vi "GL SwitchStatus.vi"(6 "error in (no error)":errorcluster, 7 "ShowWarning?":bool, 8 "Axis":T2 items=["Axis 1", "Axis 2", "Axis 3", "Axis 4", "Axis 5", "Axis 6", "Axis 7", "Axis 8"], 9 "Galil.IGalil":refnum<k7>) -> (0 "error out":errorcluster, 1 "TS Status":T1, 2 "Axis Out":T2 items=["Axis 1", "Axis 2", "Axis 3", "Axis 4", "Axis 5", "Axis 6", "Axis 7", "Axis 8"], 3 "ref out":refnum<k7>)   [LabVIEW 2022 SP3]
doc: "Sets the operation mode for an axis or vector space."
uses:
  GL Axis Control.ctl
  Command Menu.ctl
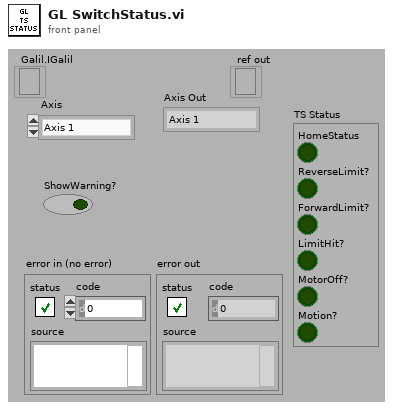
[diagram p1: front panel]
types:
  T1 = cluster{"HomeStatus":bool, "ReverseLimit?":bool, "ForwardLimit?":bool, "LimitHit?":bool, "MotorOff?":bool, "Motion?":bool}
  T2 = typedef "GL Axis Control.ctl" = u16
  T3 = typedef "Command Menu.ctl" = enum16{"CommandPassThrough", "Abort Motion", "Define Pos", "Velocity", "Acceleration", "Deceleration", "Position Rel", "Postion Abs", "Begin Move", "After Move", "Home", "KI", "KD", "KP", "IL", "Config I/O", "Set Bit", "Clear Bit", "Motor Off", "Moto On", "Status", "Execute", "Halt Execute", "HX Status", "Tell Velocity", "Check Motion", "BreakPoint", "Tell Position", "Current Code Line", "Tell Switches", "OC Force On", "OC Off", "Pos Soft Limit", "Rev Soft Limit"}
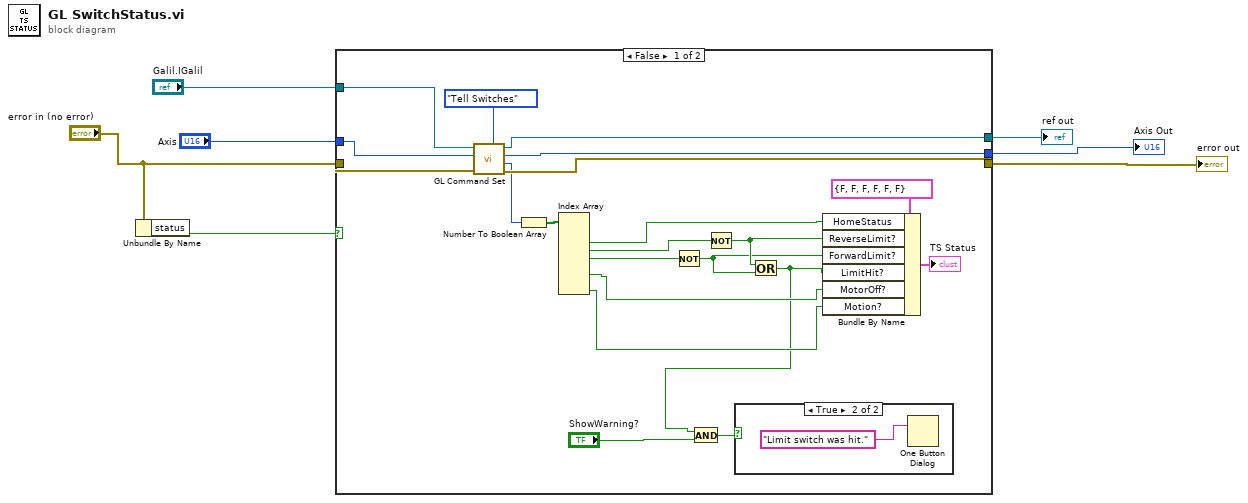
[diagram p0: block diagram]
diagram:
  n1 = Unbundle By Name("error in (no error)") -> ("status"=w5:bool)
  n2 = case shown="False" w5 {
    tunnel: "error in (no error)" -> [w26 w32]
    tunnel: [w28 w32] -> w6
    tunnel: "Galil.IGalil" -> [w14 w31]
    tunnel: "Axis" -> [w13 w30]
    tunnel: [w12 w31] -> w2
    tunnel: [w11 w30] -> w1
    frame False {
      n3 = call "GL Command Set.vi"("Command"=Command_Menu."Tell Switches", "error in (no error)"=w26, "Axis"=w13, "Galil.IGalil"=w14) -> ("error out"=w28:errorcluster, "Response#"=w25:i32, "Axis Out"=w11:T2, "ref out"=w12:refnum<k7>)  [unwired: 3 in, 1 out]
      n4 = Number To Boolean Array(number=w25) -> (Boolean array=w24:bool[])
      n5 = Index Array(array=w24) -> (element #2=w19:bool, element #3=w17:bool, element #4=w15:bool, element #6=w16:bool, element #8=w20:bool)  [unwired: 8 in, 3 out]
      n6 = Not(x=w15) -> (.not. x?=w21:bool)
      n7 = Not(x=w17) -> (.not. x?=w22:bool)
      n8 = Or(x=w22, y=w21) -> (x .or. y?=w10:bool)
      n9 = And(x=w10, y="ShowWarning?") -> (x .and. y?=w9:bool)
      n10 = case shown="True" w9 {
        frame False {
        }
        frame True {
          n11 = One Button Dialog(message="Limit switch was hit.") -> ()  [unwired: 1 in, 1 out]
        }
      }
      n12 = Bundle By Name(cluster=T1 {"HomeStatus"=FALSE, "ReverseLimit?"=FALSE, "ForwardLimit?"=FALSE, "LimitHit?"=FALSE, "MotorOff?"=FALSE, "Motion?"=FALSE}, "HomeStatus"=w19, "ReverseLimit?"=w22, "ForwardLimit?"=w21, "LimitHit?"=w10, "MotorOff?"=w16, "Motion?"=w20) -> (→"TS Status":T1)
    }
    frame True {
    }
  }
  "error out" <- w6
  "ref out" <- w2
  "Axis Out" <- w1
